vi "ChangePathToVIRefCallerDefault.vi"(4 "error in (no error)":errorcluster, 7 "VI path":path) -> (0 "error out":errorcluster, 3 "VI reference":refnum<vi>)   [LabVIEW 2020, in "NI_ReportGenerationCore.lvlib"]
uses:
  <vilib>/Utility/NIReport.llb/NI_ReportGenerationCore.lvlib
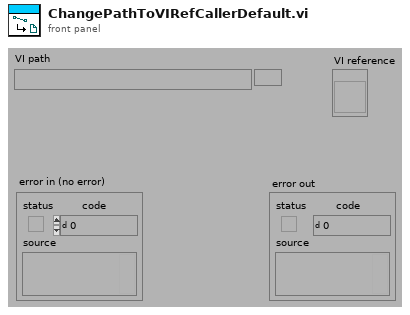
[diagram p1: front panel]
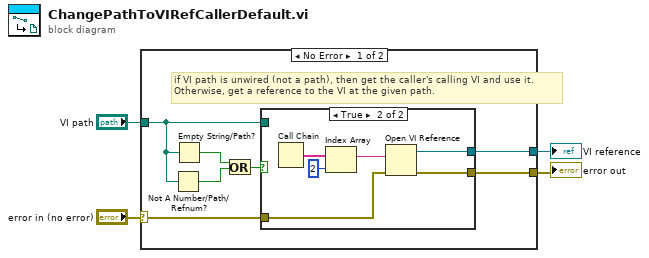
[diagram p0: block diagram]
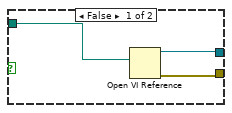
[diagram p2: hidden frame]
diagram:
  n1 = case shown="No Error" "error in (no error)" {
    selector: "error in (no error)" -> [w5 w21]
    tunnel: "VI path" -> [w11 _]
    tunnel: [w10 w21] -> w3
    tunnel: [w9 _] -> w2
    frame No Error {
      # "if VI path is unwired (not a path), then get the caller's calling VI and use it. \nOtherwise, get a reference to the VI at the given path."
      n2 = Not A Number/Path/Refnum?(number/path/refnum=w11) -> (NaN/Path/Refnum?=w7:bool)
      n3 = Empty String/Path?(string/path=w11) -> (empty?=w6:bool)
      n4 = Or(x=w6, y=w7) -> (x .or. y?=w8:bool)
      n5 = case shown="True" w8 {
        tunnel: [w13 w17] -> w9
        tunnel: [w12 w16] -> w10
        tunnel: w11 -> [w14 _]
        tunnel: w5 -> [_ w15]
        frame False {
          n6 = Open VI Reference(vi path=w14) -> (vi reference=w13:refnum<vi>, error out=w12:errorcluster)  [unwired: 5 in]
        }
        frame True {
          n7 = Call Chain() -> (call chain=w20:string[])
          n8 = Index Array(array=w20, index=2 ("Index")) -> (element=w18:string)
          n9 = Open VI Reference(vi path=w18, error in (no error)=w15) -> (vi reference=w17:refnum<vi>, error out=w16:errorcluster)  [unwired: 4 in]
        }
      }
    }
    frame Error {
    }
  }
  "error out" <- w3
  "VI reference" <- w2
